vi "Wrapper.vi"(7 "Data Map":variant, 8 "error in":errorcluster, 9 "Save?":bool, 10 "File Ref":refnum<file>, 11 "File Actor in":refnum<class "File Actor.lvclass">) -> (0 "error out":errorcluster)   [LabVIEW 2018, in "Controller.lvlib" / "Exe Write Main.lvclass"]
uses:
  Exe Write Main.lvclass
  File Actor/File Actor.lvclass
  reusable/Data/Data.lvclass
panel:
  out "Array":errorcluster[](array[cluster])
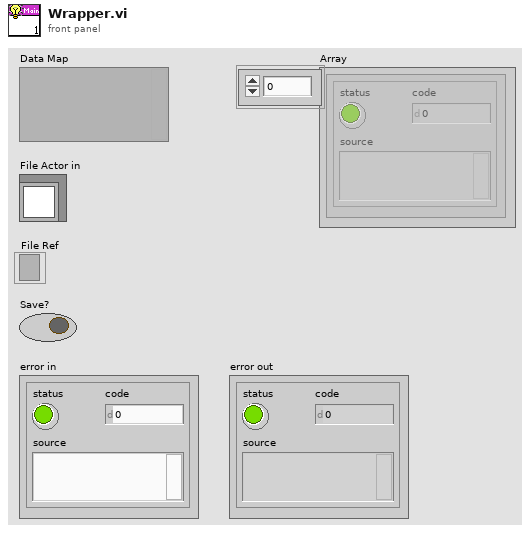
[diagram p1: front panel]
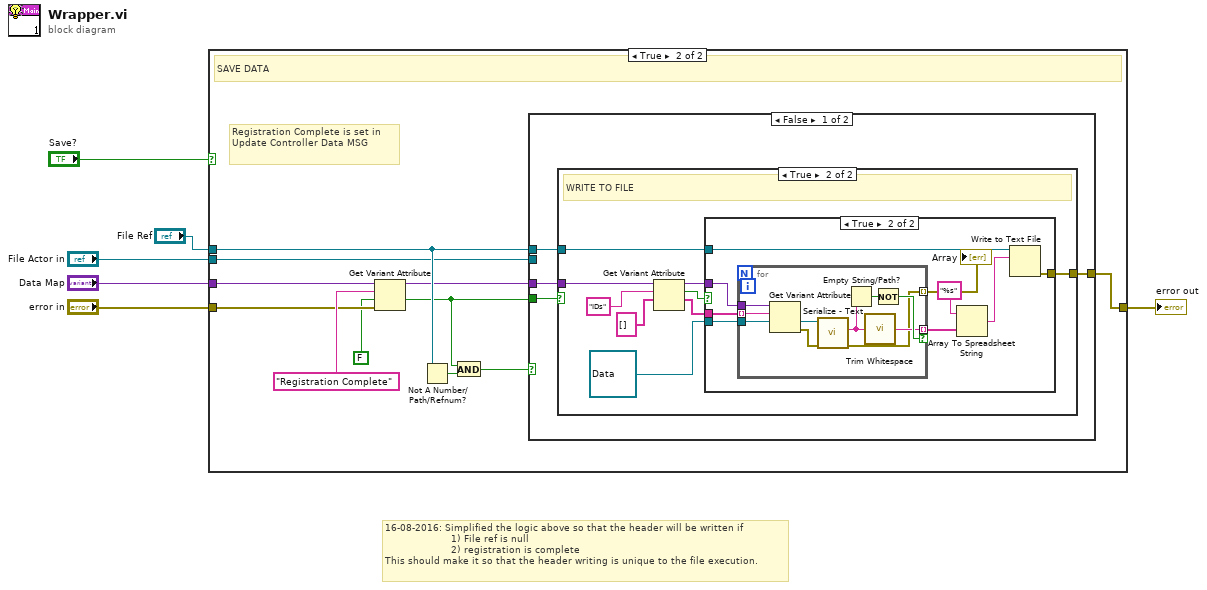
[diagram p0: block diagram]
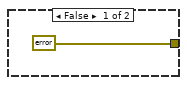
[diagram p4: hidden frame]
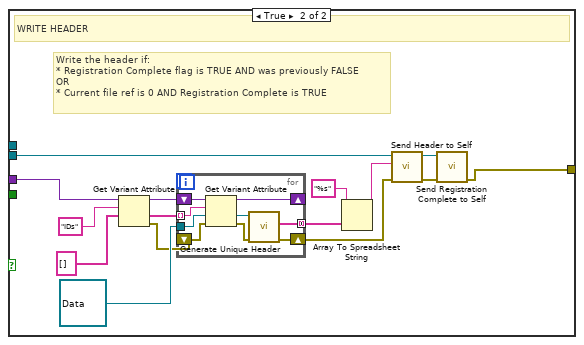
[diagram p5: hidden frame]
diagram:
  # "16-08-2016: Simplified the logic above so that the header will be written if \n                      1) File ref is null\n                      2) registration is complete\nThis should make it so that the header writing is unique to the file execution."
  n1 = case shown="True" "Save?" {
    tunnel: [w7 w18] -> w6
    tunnel: "File Ref" -> [_ w15]
    tunnel: "error in" -> [w7 w12]
    tunnel: "Data Map" -> [_ w17]
    tunnel: "File Actor in" -> [_ w11]
    frame False {
      # "NO SAVE"
    }
    frame True {
      # "Registration Complete is set in Update Controller Data MSG"
      # "SAVE DATA"
      n2 = Get Variant Attribute(Variant=w17, name="Registration Complete", default value (empty Variant)=FALSE, error in=w12) -> (duplicate Variant=w10:variant, value=w13:bool)  [unwired: 2 out]
      n3 = Not A Number/Path/Refnum?(number/path/refnum=w15) -> (NaN/Path/Refnum?=w14:bool)
      n4 = And(x=w13, y=w14) -> (x .and. y?=w8:bool)
      n5 = case shown="False" w8 {
        tunnel: [w22 w66] -> w18
        tunnel: w15 -> [w21 _]
        tunnel: w10 -> [w20 w65]
        tunnel: w13 -> [w19 _]
        tunnel: w11 -> [_ w57]
        frame False {
          n6 = case shown="True" w19 {
            tunnel: [_ w31] -> w22
            tunnel: w21 -> [_ w29]
            tunnel: w20 -> [_ w30]
            frame False {
            }
            frame True {
              # "WRITE TO FILE"
              n7 = Get Variant Attribute(Variant=w30, name="IDs", default value (empty Variant)=string[] []) -> (duplicate Variant=w24:variant, found=w25:bool, value=w26:string[])  [unwired: 1 in, 1 out]
              n8 = case shown="True" w25 {
                tunnel: w26 -> [_ w41]
                tunnel: w24 -> [_ w40]
                tunnel: refnum<class "Data.lvclass"> refnum ("Base Data Lib:Data") -> [_ w39]
                tunnel: w29 -> [_ w36]
                tunnel: [errorcluster {"status"=FALSE, "code"=0, "source"=""} ("error out") w35] -> w31
                frame False {
                }
                frame True {
                  n9 = for {
                    tunnel: w41 -> [w43] mode=indexing
                    tunnel: w40 -> [w51]
                    tunnel: w39 -> [w50]
                    tunnel: [w44] -> w38 mode=indexing if=w46
                    tunnel: [w42] -> w33 mode=indexing
                    n10 = Get Variant Attribute(Variant=w51, name=w43, default value (empty Variant)=w50) -> (value=w49:refnum<class "Data.lvclass">, error out=w48:errorcluster)  [unwired: 1 in, 2 out]
                    n11 = call-dynamic "Serialize - Text.vi"("error in"=w48, "Data in"=w49) -> ("error out"=w42:errorcluster, "Serialized Text"=w45:string)  [unwired: 7 in, 1 out]
                    n12 = Empty String/Path?(string/path=w45) -> (empty?=w47:bool)
                    n13 = call <vilib>:"Trim Whitespace.vi"("string"=w45) -> ("trimmed string"=w44:string)  [unwired: 1 in]
                    n14 = Not(x=w47) -> (.not. x?=w46:bool)
                  }
                  "Array" <- w33
                  n15 = Array To Spreadsheet String(array=w38, 3:"%s" ("format string")) -> (spreadsheet string=w34:string)  [unwired: 1 in]
                  n16 = Write to Text File(file (use dialog)=w36, text=w34) -> (error out=w35:errorcluster)  [unwired: 2 in, 2 out]
                }
              }
            }
          }
        }
        frame True {
          # "Write the header if:\n* Registration Complete flag is TRUE AND was previously FALSE\nOR \n* Current file ref is 0 AND Registration Complete is TRUE"
          # "WRITE HEADER"
          n17 = Get Variant Attribute(Variant=w65, name="IDs", default value (empty Variant)=string[] []) -> (duplicate Variant=w61:variant, value=w62:string[], error out=w53:errorcluster)  [unwired: 1 in, 1 out]
          n18 = for {
            tunnel: w62 -> [w75] mode=indexing
            tunnel: refnum<class "Data.lvclass"> refnum ("Base Data Lib:Data") -> [w73]
            tunnel: [w71] -> w59 mode=concatenating
            shift-right: [w68] -> w52
            shift-left: w53 -> [w69]
            shift-right: [w67] -> _
            shift-left: w61 -> [w74]
            n19 = Get Variant Attribute(Variant=w74, name=w75, default value (empty Variant)=w73, error in=w69) -> (duplicate Variant=w67:variant, value=w72:refnum<class "Data.lvclass">, error out=w70:errorcluster)  [unwired: 1 out]
            n20 = call-dynamic "Generate Unique Header.vi"("error in"=w70, "Data in"=w72) -> ("error out"=w68:errorcluster, "Header"=w71:string[])  [unwired: 7 in, 1 out]
          }
          n21 = Array To Spreadsheet String(array=w59, 3:"%s" ("format string")) -> (spreadsheet string=w55:string)  [unwired: 1 in]
          n22 = call "Send Header to Self.vi"("error in"=w52, "Header"=w55, "File Actor in"=w57) -> ("error out"=w54:errorcluster, "File Actor out"=w56:refnum<class "File Actor.lvclass">)  [unwired: 7 in]
          n23 = call "Send Registration Complete to Self.vi"("error in (no error)"=w54, "File Actor in"=w56) -> ("error out"=w66:errorcluster)  [unwired: 8 in, 1 out]
        }
      }
    }
  }
  "error out" <- w6
